vi "checkIfBusy.vi"(8 "error in (no error)":errorcluster, 11 "Monochromator in":refnum<class "Monochromator.lvclass">) -> (0 "error out":errorcluster, 3 "Monochromator out":refnum<class "Monochromator.lvclass">)   [LabVIEW 2016, in "Monochromator.lvclass"]
uses:
  Monochromator.lvclass
  Monochromator.lvclass/Monochromator.ctl
  MonoStates/MonoState/MonoState.lvclass
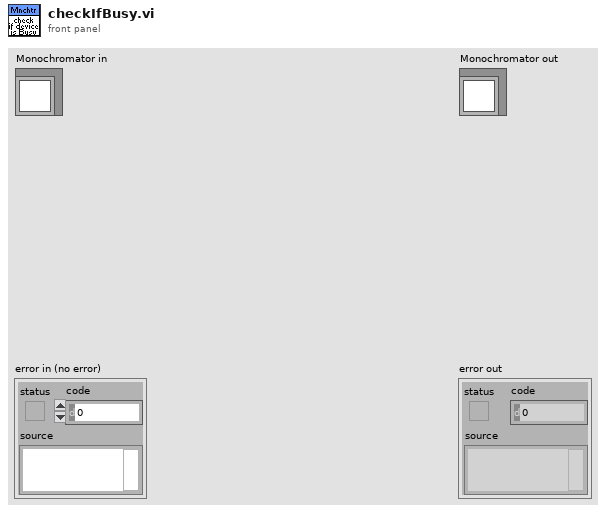
[diagram p1: front panel]
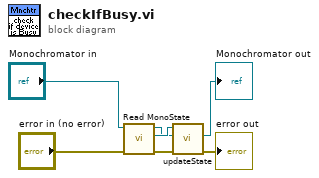
[diagram p0: block diagram]
diagram:
  n1 = call "Read MonoState.vi"("error in (no error)"="error in (no error)", "Monochromator in"="Monochromator in") -> ("error out"=w1:errorcluster, "MonoState.lvclass"=w3:refnum<class "MonoState.lvclass">, "Monochromator out"=w2:refnum<class "Monochromator.lvclass">)  [unwired: 7 in]
  n2 = call-dynamic "updateState.vi"("error in (no error)"=w1, "Monochromator in"=w2, "MonoState in"=w3) -> ("error out"=→"error out":errorcluster, "Monochromator out"=→"Monochromator out":refnum<class "Monochromator.lvclass">)  [unwired: 6 in, 1 out]
